vi "Year2019 Q5.vi"() -> ()   [LabVIEW 2018]
panel:
  out "XY Graph":cluster{dbl[], dbl[]}[](graph)
  in  "Radius r":dbl
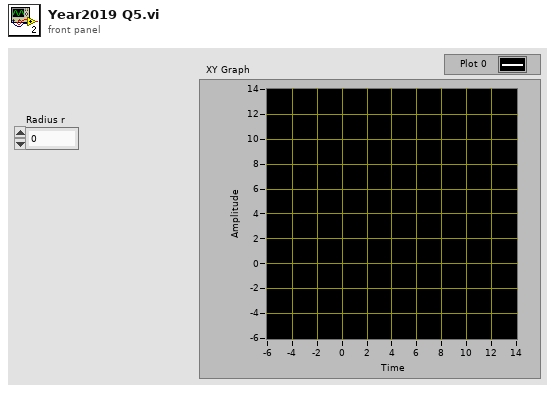
[diagram p1: front panel]
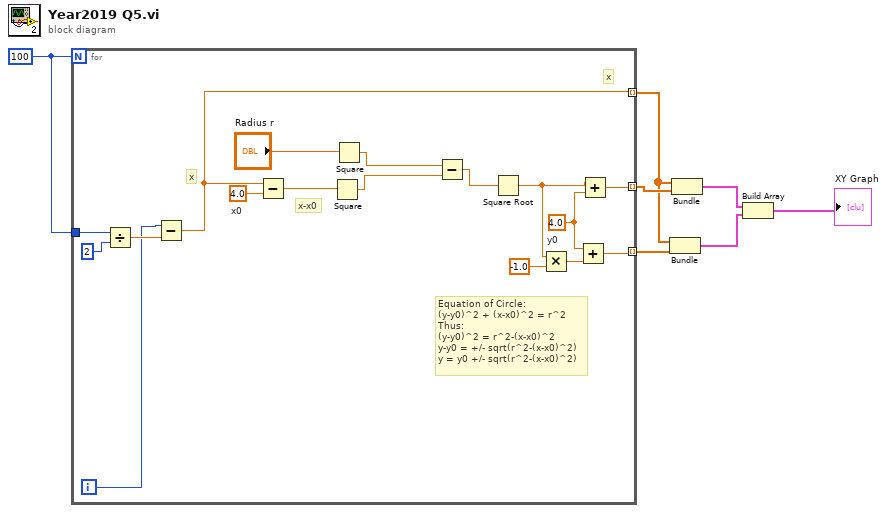
[diagram p0: block diagram]
diagram:
  w6 = 100
  n1 = for {
    N: w6 -> [_]
    tunnel: [w12] -> w7 mode=indexing
    tunnel: w6 -> [w23]
    tunnel: [w18] -> w5 mode=indexing
    tunnel: [w10] -> w4 mode=indexing
    i -> [w20]
    w8 = 4.0  # y0
    w17 = 4.0  # x0
    # "Equation of Circle:\n(y-y0)^2 + (x-x0)^2 = r^2\nThus:\n(y-y0)^2 = r^2-(x-x0)^2\ny-y0 = +/- sqrt(r^2-(x-x0)^2)\ny = y0 +/- sqrt(r^2-(x-x0)^2)"
    # "x-x0"
    # "x"
    # "x"
    n2 = Divide(x=w23, y=2) -> (x/y=w21:dbl)
    n3 = Subtract(x=w20, y=w21) -> (x-y=w18:dbl)
    n4 = Subtract(x=w18, y=w17) -> (x-y=w16:dbl)
    n5 = Square(x=w16) -> (x^2=w14:dbl)
    n6 = Square(x="Radius r") -> (x^2=w15:dbl)
    n7 = Subtract(x=w15, y=w14) -> (x-y=w13:dbl)
    n8 = Square Root(x=w13) -> (sqrt(x)=w9:dbl)
    n9 = Multiply(x=w9, y=-1.0) -> (x*y=w11:dbl)
    n10 = Add(x=w8, y=w11) -> (x+y=w10:dbl)
    n11 = Add(x=w9, y=w8) -> (x+y=w12:dbl)
  }
  n12 = Bundle "Bundle"(w5, w4) -> (w2:cluster{dbl[], dbl[]})  [unwired: 1 in]
  n13 = Bundle "Bundle"(w5, w7) -> (w3:cluster{dbl[], dbl[]})  [unwired: 1 in]
  n14 = Build Array "Build Array"(w3, w2) -> (→"XY Graph":cluster{dbl[], dbl[]}[])
